vi "Get_Coordinates.vi"(4 "Error in":errorcluster, 6 "Longitude in":sgl caption="Longitude", 7 "Latitude in":sgl caption="Latitude") -> (0 "Error out":errorcluster, 1 "Not equal?":bool, 2 "Longitude out":sgl, 3 "Latitude out":sgl)   [LabVIEW 2013]
uses:
  VantagePro.dll
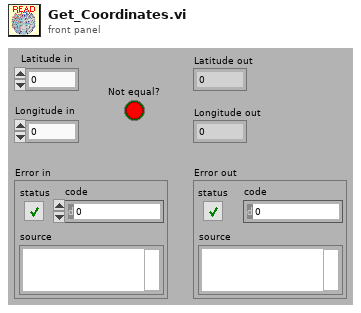
[diagram p1: front panel]
types:
  T1 = cluster{"bUsefractdegr":i16, "dummy1":i8, "dummy2":i8, "fractiondegr":sgl, "bNegdegrees":i16, "degrees":i16, "minutes":i16, "seconds":i16}
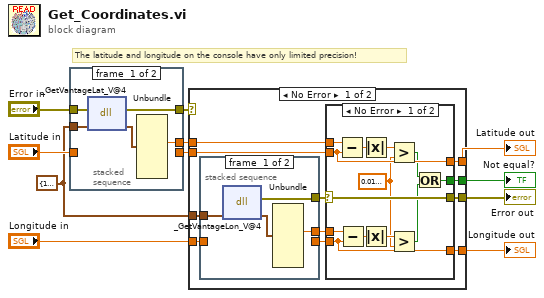
[diagram p0: block diagram]
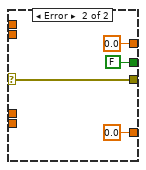
[diagram p2: hidden frame]
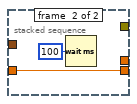
[diagram p3: hidden frame]
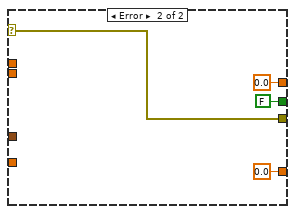
[diagram p4: hidden frame]
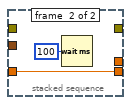
[diagram p5: hidden frame]
diagram:
  w1 = T1 {"bUsefractdegr"=1, "dummy1"=0, "dummy2"=0, "fractiondegr"=0.0, "bNegdegrees"=0, "degrees"=0, "minutes"=0, "seconds"=0}
  # "The latitude and longitude on the console have only limited precision!"
  n1 = stacked-sequence {
    tunnel: "Latitude in" -> [_ w17]
    tunnel: [_ w17] -> w7
    tunnel: w1 -> [w16 _]
    tunnel: [w14 _] -> w8
    tunnel: [w13 _] -> w10
    tunnel: "Error in" -> [w12 _]
    frame #0 {
      n2 = dll-call lib="C:/Users/Bob van Eijk/Desktop/LabView Projects 13/HiSPARC Weather Station/Develop/VantagePro.dll" fn="_GetVantageLat_V@4" label="Get latitude"(error in=w12, "latitude"=w16) -> (error out=w13:errorcluster, "latitude"=w15:T1)  [unwired: 3 in, 1 out]
      n3 = Unbundle(w15) -> ("fractiondegr"=w14:sgl)  [unwired: 7 out]
    }
    frame #1 {
      n4 = Wait (ms)(milliseconds to wait=u32 100) -> ()  [unwired: 1 out]
    }
  }
  n5 = case shown="No Error" w10 {
    selector: w10 -> [_ w56]
    tunnel: "Longitude in" -> [w29 _]
    tunnel: w1 -> [w28 _]
    tunnel: w8 -> [w25 _]
    tunnel: w7 -> [w24 _]
    tunnel: [w22 FALSE] -> w2
    tunnel: [w21 w56] -> w6
    tunnel: [w20 sgl 0.0] -> w3
    tunnel: [w19 sgl 0.0] -> w4
    frame No Error {
      n6 = stacked-sequence {
        tunnel: w29 -> [_ w51]
        tunnel: [_ w51] -> w23
        tunnel: [w50 _] -> w27
        tunnel: w28 -> [w48 _]
        tunnel: [w47 _] -> w26
        frame #0 {
          n7 = dll-call lib="C:/Users/Bob van Eijk/Desktop/LabView Projects 13/HiSPARC Weather Station/Develop/VantagePro.dll" fn="_GetVantageLon_V@4" label="Get longitude"(w48) -> (error out=w50:errorcluster, w49:T1)  [unwired: 4 in, 1 out]
          n8 = Unbundle(w49) -> ("fractiondegr"=w47:sgl)  [unwired: 7 out]
        }
        frame #1 {
          n9 = Wait (ms)(milliseconds to wait=u32 100) -> ()  [unwired: 1 out]
        }
      }
      n10 = case shown="No Error" w27 {
        selector: w27 -> [w41 w46]
        tunnel: w26 -> [w33 _]
        tunnel: w25 -> [w38 _]
        tunnel: w24 -> [w37 _]
        tunnel: w23 -> [w32 _]
        tunnel: [w42 FALSE] -> w22
        tunnel: [w41 w46] -> w21
        tunnel: [w32 sgl 0.0] -> w20
        tunnel: [w37 sgl 0.0] -> w19
        frame No Error {
          w30 = sgl 0.02
          n11 = Subtract(x=w38, y=w37) -> (x-y=w39:sgl)
          n12 = Subtract(x=w33, y=w32) -> (x-y=w34:sgl)
          n13 = Absolute Value(x=w39) -> (abs(x)=w40:sgl)
          n14 = Absolute Value(x=w34) -> (abs(x)=w35:sgl)
          n15 = Greater?(x=w40, y=w30) -> (0:w36:bool)
          n16 = Greater?(x=w35, y=w30) -> (0:w31:bool)
          n17 = Or(x=w36, y=w31) -> (x .or. y?=w42:bool)
        }
        frame Error {
        }
      }
    }
    frame Error {
    }
  }
  "Error out" <- w6
  "Latitude out" <- w4
  "Longitude out" <- w3
  "Not equal?" <- w2
